vi "Write Data Frame Options.vi"(7 "Unit ID (A)":string="A", 8 "error in":errorcluster, 9 "Enables: Data frame only":T2={"Valve Drive"=FALSE, "Totalizer"=TRUE, "Totalizer Timer"=FALSE, "Totalizer Peak Flow"=FALSE, "Show Abs., Gauge\nand Baro. pressures"=FALSE}, 10 "Enables: \nData frame and Display":T1={"Pressure(s)"=TRUE, "Temperature"=TRUE, "Volumetric"=TRUE, "Mass"=TRUE, "Totalizer Average Flow"=FALSE, "Gas Selected"=TRUE}, 11 "VISA Session In":refnum<visa-resource-name>="Alicat") -> (0 "error out":errorcluster, 3 "VISA Session Out":refnum<visa-resource-name>)   [LabVIEW 2020]
doc: "Writes new options into an Alicat device to modify the data frame output. This can be used to pare down an Alicat's data frame to increase the serial data speed."
panel:
  # "Some features may not be possible to enable/disable.\nThis depends on the software version and device type.\nIf unable to enable/disable, the changes will not take."
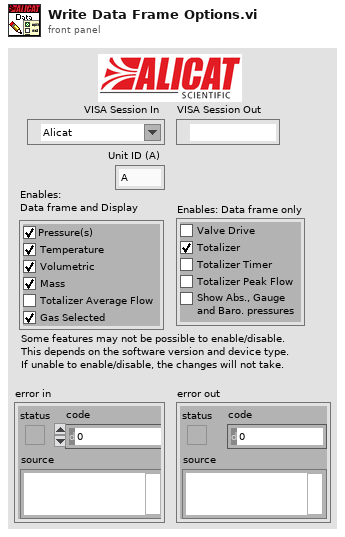
[diagram p1: front panel]
types:
  T1 = cluster{"Pressure(s)":bool, "Temperature":bool, "Volumetric":bool, "Mass":bool, "Totalizer Average Flow":bool, "Gas Selected":bool}
  T2 = cluster{"Valve Drive":bool, "Totalizer":bool, "Totalizer Timer":bool, "Totalizer Peak Flow":bool, "Show Abs., Gauge\nand Baro. pressures":bool}
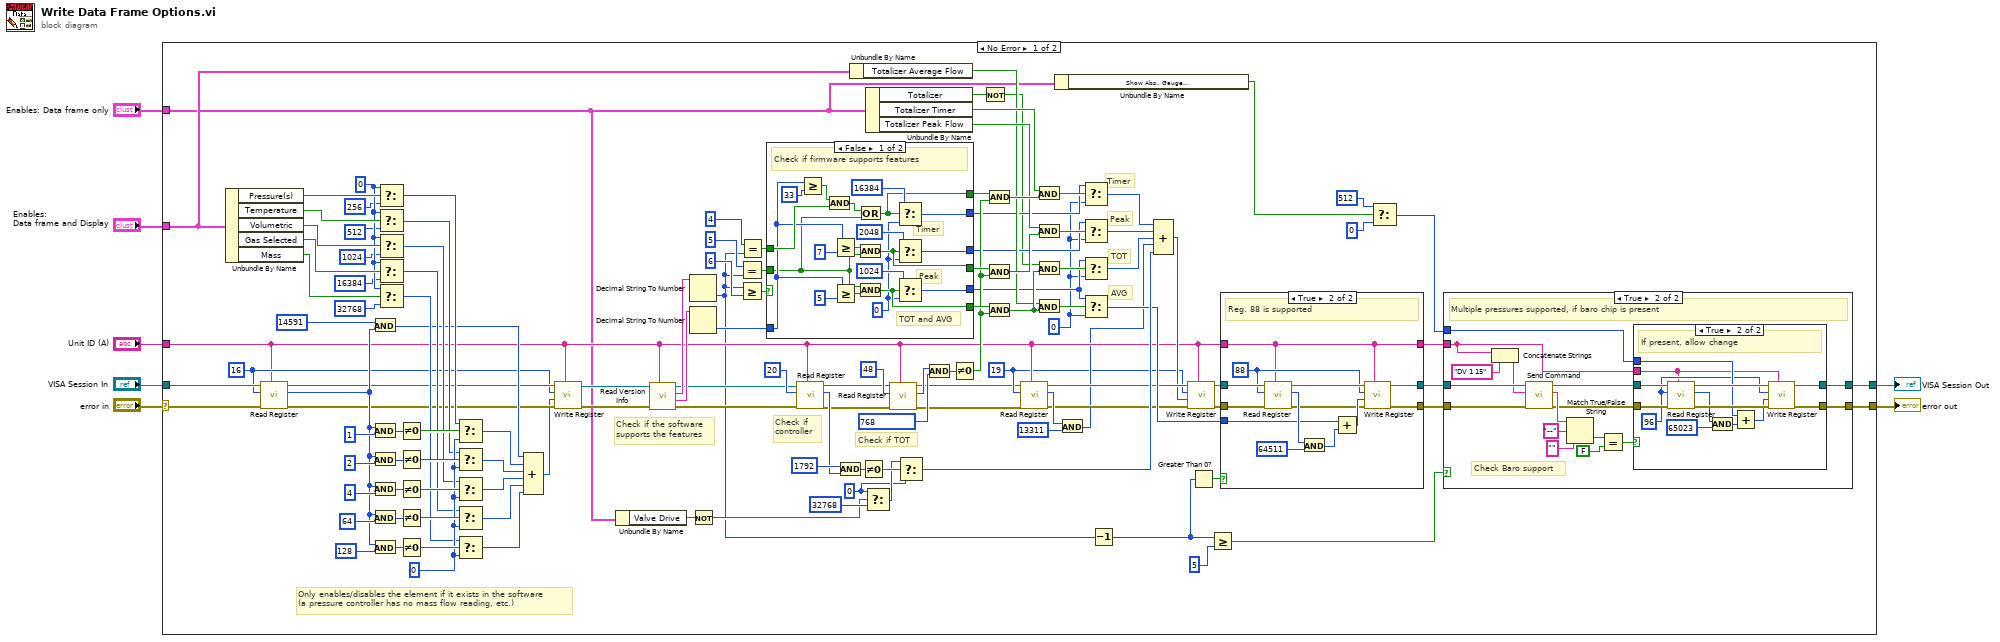
[diagram p0: block diagram]
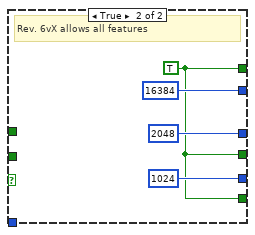
[diagram p5: hidden frame]
diagram:
  n1 = case shown="No Error" "error in" {
    selector: "error in" -> [w124 w209]
    tunnel: "VISA Session In" -> [w135 w210]
    tunnel: "Unit ID (A)" -> [w29 _]
    tunnel: [w10 w210] -> w7
    tunnel: [w11 w209] -> w6
    tunnel: "Enables: \nData frame and Display" -> [w89 _]
    tunnel: "Enables: Data frame only" -> [w9 _]
    frame No Error {
      w40 = 0 ("f")
      w80 = 0 ("f")
      w27 = u16 19 ("Register address")
      w106 = 0 ("Register Value (U16)")
      w113 = 0 ("Register Value (U16)")
      w91 = u16 16 ("Register address")
      # "AVG"
      # "TOT"
      # "Peak"
      # "Timer"
      # "Check if TOT"
      # "Check if the software\nsupports the features"
      # "Check if\ncontroller"
      # "Only enables/disables the element if it exists in the software\n(a pressure controller has no mass flow reading, etc.)"
      n2 = Unbundle By Name(w89) -> ("Pressure(s)"=w118:bool, "Temperature"=w117:bool, "Volumetric"=w116:bool, "Gas Selected"=w115:bool, "Mass"=w114:bool)
      n3 = call "Read Register.vi"("Unit ID (A)"=w29, "error in"=w124, "Register address"=w91, "VISA Session In"=w135) -> ("error out"=w93:errorcluster, "Register Value (I32)"=w100:i32, "VISA Session Out"=w92:refnum<visa-resource-name>)  [unwired: 5 in]
      n4 = And(x=14591, y=w100) -> (x .and. y?=w99:i32)
      n5 = And(x=w100, y=1 ("Register Value (U16)")) -> (x .and. y?=w130:i32)
      n6 = And(x=w100, y=2 ("Register Value (U16)")) -> (x .and. y?=w129:i32)
      n7 = And(x=w100, y=4 ("Register Value (U16)")) -> (x .and. y?=w128:i32)
      n8 = And(x=w100, y=64 ("Register Value (U16)")) -> (x .and. y?=w127:i32)
      n9 = And(x=w100, y=128 ("Register Value (U16)")) -> (x .and. y?=w125:i32)
      n10 = Select(t=w113, s=w118, f=256 ("Register Value (U16)")) -> (s? t:f=w107:i32)
      n11 = Select(t=w113, s=w117, f=512 ("Register Value (U16)")) -> (s? t:f=w105:i32)
      n12 = Select(t=w113, s=w116, f=1024 ("Register Value (U16)")) -> (s? t:f=w104:i32)
      n13 = Select(t=w113, s=w115, f=16384 ("Register Value (U16)")) -> (s? t:f=w103:i32)
      n14 = Select(t=w113, s=w114, f=32768 ("Register Value (U16)")) -> (s? t:f=w102:i32)
      n15 = Not Equal To 0?(x=w130) -> (x != 0?=w123:bool)
      n16 = Not Equal To 0?(x=w129) -> (x != 0?=w122:bool)
      n17 = Not Equal To 0?(x=w128) -> (x != 0?=w121:bool)
      n18 = Not Equal To 0?(x=w127) -> (x != 0?=w120:bool)
      n19 = Not Equal To 0?(x=w125) -> (x != 0?=w119:bool)
      n20 = Select(t=w107, s=w123, f=w106) -> (s? t:f=w98:i32)
      n21 = Select(t=w105, s=w122, f=w106) -> (s? t:f=w94:i32)
      n22 = Select(t=w104, s=w121, f=w106) -> (s? t:f=w95:i32)
      n23 = Select(t=w103, s=w120, f=w106) -> (s? t:f=w96:i32)
      n24 = Select(t=w102, s=w119, f=w106) -> (s? t:f=w97:i32)
      n25 = Compound Arithmetic op=ADD(w99, w98, w94, w95, w96, w97) -> (w90:i32)
      n26 = call "Write Register.vi"("Unit ID (A)"=w29, "error in"=w93, "Register Value"=w90, "Register address"=w91, "VISA Session In"=w92) -> ("error out"=w60:errorcluster, "VISA Session Out"=w61:refnum<visa-resource-name>)  [unwired: 4 in, 1 out]
      n27 = Unbundle By Name(w9) -> ("Valve Drive"=w63:bool)
      n28 = call "Read Version Info.vi"("Unit ID (A)"=w29, "error in"=w60, "VISA Session In"=w61) -> ("error out"=w65:errorcluster, "Software Sub-Rev"=w74:string, "Software Rev"=w75:string, "VISA Session Out"=w64:refnum<visa-resource-name>)  [unwired: 4 in, 1 out]
      n29 = Decimal String To Number(string=w75) -> (number=w21:i32)  [unwired: 2 in, 1 out]
      n30 = Decimal String To Number(string=w74) -> (number=w67:i32)  [unwired: 2 in, 1 out]
      n31 = Not(x=w63) -> (.not. x?=w62:bool)
      n32 = Equal?(x=5 ("y"), y=w21) -> (x = y?=w66:bool)
      n33 = Greater Or Equal?(x=w21, y=6) -> (x >= y?=w69:bool)
      n34 = Equal?(x=4 ("y"), y=w21) -> (x = y?=w68:bool)
      n35 = case shown="False" w69 {
        tunnel: w68 -> [w203 _]
        tunnel: w67 -> [w195 _]
        tunnel: w66 -> [w193 _]
        tunnel: [w192 w205] -> w55
        tunnel: [w191 w205] -> w57
        tunnel: [w190 w205] -> w56
        tunnel: [w188 16384 ("Register Value (U16)")] -> w43
        tunnel: [w187 2048 ("Register Value (U16)")] -> w42
        tunnel: [w186 1024 ("Register Value (U16)")] -> w41
        frame False {
          w185 = 0 ("Register Value (U16)")
          # "Timer"
          # "Peak"
          # "TOT and AVG"
          # "Check if firmware supports features"
          n36 = Greater Or Equal?(x=w195, y=33 ("x")) -> (x >= y?=w204:bool)
          n37 = And(x=w204, y=w203) -> (x .and. y?=w201:bool)
          n38 = Greater Or Equal?(x=w195, y=7 ("x")) -> (x >= y?=w198:bool)
          n39 = Greater Or Equal?(x=w195, y=5 ("x")) -> (x >= y?=w194:bool)
          n40 = Or(x=w201, y=w193) -> (x .or. y?=w191:bool)
          n41 = And(x=w198, y=w193) -> (x .and. y?=w192:bool)
          n42 = And(x=w193, y=w194) -> (x .and. y?=w190:bool)
          n43 = Select(t=16384 ("Register Value (U16)"), s=w191, f=w185) -> (s? t:f=w188:i32)
          n44 = Select(t=2048 ("Register Value (U16)"), s=w192, f=w185) -> (s? t:f=w187:i32)
          n45 = Select(t=1024 ("Register Value (U16)"), s=w190, f=w185) -> (s? t:f=w186:i32)
        }
        frame True {
          w205 = TRUE
          # "Rev. 6vX allows all features"
        }
      }
      n46 = call "Read Register.vi"("Unit ID (A)"=w29, "error in"=w65, "Register address"=u16 20, "VISA Session In"=w64) -> ("error out"=w58:errorcluster, "Register Value (I32)"=w85:i32, "VISA Session Out"=w59:refnum<visa-resource-name>)  [unwired: 5 in]
      n47 = And(x=1792 ("Register Value (U16)"), y=w85) -> (x .and. y?=w86:i32)
      n48 = Unbundle By Name(w89) -> ("Totalizer Average Flow"=w48:bool)
      n49 = Not Equal To 0?(x=w86) -> (x != 0?=w82:bool)
      n50 = Select(t=w80, s=w62, f=32768 ("Register Value (U16)")) -> (s? t:f=w81:i32)
      n51 = Unbundle By Name(w9) -> ("Totalizer"=w30:bool, "Totalizer Timer"=w52:bool, "Totalizer Peak Flow"=w49:bool)
      n52 = call "Read Register.vi"("Unit ID (A)"=w29, "error in"=w58, "Register address"=u16 48, "VISA Session In"=w59) -> ("error out"=w24:errorcluster, "Register Value (I32)"=w77:i32, "VISA Session Out"=w23:refnum<visa-resource-name>)  [unwired: 5 in]
      n53 = Select(t=w81, s=w82, f=w80) -> (s? t:f=w36:i32)
      n54 = And(x=w77, y=768) -> (x .and. y?=w76:i32)
      n55 = Not Equal To 0?(x=w76) -> (x != 0?=w54:bool)
      n56 = Not(x=w30) -> (.not. x?=w31:bool)
      n57 = And(x=w57, y=w54) -> (x .and. y?=w53:bool)
      n58 = And(x=w55, y=w54) -> (x .and. y?=w50:bool)
      n59 = And(x=w56, y=w54) -> (x .and. y?=w51:bool)
      n60 = call "Read Register.vi"("Unit ID (A)"=w29, "error in"=w24, "Register address"=w27, "VISA Session In"=w23) -> ("error out"=w34:errorcluster, "Register Value (I32)"=w73:i32, "VISA Session Out"=w33:refnum<visa-resource-name>)  [unwired: 5 in]
      n61 = And(x=w52, y=w53) -> (x .and. y?=w45:bool)
      n62 = And(x=w49, y=w50) -> (x .and. y?=w44:bool)
      n63 = And(x=w31, y=w51) -> (x .and. y?=w46:bool)
      n64 = And(x=w48, y=w51) -> (x .and. y?=w47:bool)
      n65 = Unbundle By Name(w9) -> ("Show Abs., Gauge\nand Baro. pressures"=w8:bool)
      n66 = And(x=w73, y=13311 ("Register Value (U16)")) -> (x .and. y?=w28:i32)
      n67 = Select(t=w43, s=w45, f=w40) -> (s? t:f=w39:i32)
      n68 = Select(t=w42, s=w44, f=w40) -> (s? t:f=w38:i32)
      n69 = Select(t=w41, s=w46, f=w40) -> (s? t:f=w37:i32)
      n70 = Select(t=w41, s=w47, f=w40) -> (s? t:f=w35:i32)
      n71 = Decrement(x=w21) -> (x-1=w20:i32)
      n72 = Compound Arithmetic op=ADD(w39, w38, w37, w28, w36) -> (w32:i32)
      n73 = call "Write Register.vi"("Unit ID (A)"=w29, "error in"=w34, "Register Value"=w32, "Register address"=w27, "VISA Session In"=w33) -> ("error out"=w26:errorcluster, "VISA Session Out"=w25:refnum<visa-resource-name>)  [unwired: 4 in, 1 out]
      n74 = Greater Than 0?(x=w20) -> (x > 0?=w22:bool)
      n75 = Greater Or Equal?(x=w20, y=5) -> (x >= y?=w18:bool)
      n76 = case shown="True" w22 {
        tunnel: w35 -> [_ w181]
        tunnel: [w170 w179] -> w16
        tunnel: [w171 w178] -> w17
        tunnel: w29 -> [w169 w172]
        tunnel: w26 -> [w170 w177]
        tunnel: w25 -> [w171 w174]
        tunnel: [w169 w172] -> w15
        frame False {
          # "Board rev 21 and below dont support this"
        }
        frame True {
          w173 = u16 88 ("Register address")
          # "Reg. 88 is supported"
          n77 = call "Read Register.vi"("Unit ID (A)"=w172, "error in"=w177, "Register address"=w173, "VISA Session In"=w174) -> ("error out"=w176:errorcluster, "Register Value (I32)"=w183:i32, "VISA Session Out"=w175:refnum<visa-resource-name>)  [unwired: 5 in]
          n78 = And(x=w183, y=64511 ("Register Value (U16)")) -> (x .and. y?=w182:i32)
          n79 = Add(x=w181, y=w182) -> (x+y=w180:i32)
          n80 = call "Write Register.vi"("Unit ID (A)"=w172, "error in"=w176, "Register Value"=w180, "Register address"=w173, "VISA Session In"=w175) -> ("error out"=w179:errorcluster, "VISA Session Out"=w178:refnum<visa-resource-name>)  [unwired: 4 in, 1 out]
        }
      }
      n81 = Select(t=512 ("y"), s=w8, f=0 ("y")) -> (s? t:f=w12:i32)
      n82 = case shown="True" w18 {
        tunnel: w17 -> [w137 w153]
        tunnel: w16 -> [w136 w152]
        tunnel: w15 -> [_ w141]
        tunnel: w12 -> [_ w140]
        tunnel: [w136 w139] -> w11
        tunnel: [w137 w138] -> w10
        frame False {
          # "Not supported"
        }
        frame True {
          # "Check Baro support"
          # "Multiple pressures supported, if baro chip is present"
          n83 = Concatenate Strings(w141, "DV 1 15" ("Command")) -> (w150:string)
          n84 = call "Send Command.vi"("error in"=w152, "Command"=w150, "VISA Session In"=w153) -> ("error out"=w143:errorcluster, "Response"=w149:string, "VISA Session Out"=w142:refnum<visa-resource-name>)  [unwired: 6 in]
          n85 = Match True/False String(2:"" ("false string"), 3:"--" ("true string"), 4:w149) -> (0:w146:bool)  [unwired: 1 out]
          n86 = Equal?(x=w146, y=FALSE) -> (x = y?=w144:bool)
          n87 = case shown="True" w144 {
            tunnel: w143 -> [w155 w167]
            tunnel: w142 -> [w154 w168]
            tunnel: w141 -> [_ w156]
            tunnel: w140 -> [_ w161]
            tunnel: [w155 w158] -> w139
            tunnel: [w154 w157] -> w138
            frame False {
              # "Not supported"
            }
            frame True {
              w159 = u16 96 ("Register address")
              # "If present, allow change"
              n88 = call "Read Register.vi"("Unit ID (A)"=w156, "error in"=w167, "Register address"=w159, "VISA Session In"=w168) -> ("error out"=w166:errorcluster, "Register Value (I32)"=w164:i32, "VISA Session Out"=w165:refnum<visa-resource-name>)  [unwired: 5 in]
              n89 = And(x=w164, y=65023) -> (x .and. y?=w162:i32)
              n90 = Add(x=w161, y=w162) -> (x+y=w160:i32)
              n91 = call "Write Register.vi"("Unit ID (A)"=w156, "error in"=w166, "Register Value"=w160, "Register address"=w159, "VISA Session In"=w165) -> ("error out"=w158:errorcluster, "VISA Session Out"=w157:refnum<visa-resource-name>)  [unwired: 4 in, 1 out]
            }
          }
        }
      }
    }
    frame Error {
    }
  }
  "error out" <- w6
  "VISA Session Out" <- w7
